vi "Write Configuration.vi"(8 "error in (no error)":errorcluster, 9 "Name (empty: type name)":string, 10 "Type":variant, 11 "ConfigurableActor in":refnum<class "ConfigurableActor.lvclass">) -> (0 "error out":errorcluster, 3 "ConfigurableActor out":refnum<class "ConfigurableActor.lvclass">)   [LabVIEW 2014, in "ConfigurableActor.lvclass"]
uses:
  ConfigurableActor.lvclass
  ConfigurableActor.lvclass/ConfigurableActor.ctl
  <vilib>/LabVIEW Open Source/Configuration Manager/Manager/ConfigManager.lvclass/ConfigManager.ctl
  <vilib>/LabVIEW Open Source/Configuration Manager/Manager/Write.vi
  <vilib>/LabVIEW Open Source/Configuration Manager/Manager/Read Serializer.vi
  <vilib>/LabVIEW Open Source/Configuration Manager/Manager/Read Encoding.vi
  <vilib>/LabVIEW Open Source/Configuration Manager/Manager/Read Encryption.vi
  <vilib>/LabVIEW Open Source/Configuration Manager/Manager/Decompose KVPs.vi
  <vilib>/Utility/VariantDataType/GetTypeInfo.vi
  <vilib>/LabVIEW Open Source/Configuration Manager/Cache/ConfigManager.Cache.lvclass
  <vilib>/LabVIEW Open Source/Configuration Manager/Manager/ConfigManager.lvclass
  <vilib>/LabVIEW Open Source/Configuration Manager/Serializer/Serializer.lvclass
  <vilib>/LabVIEW Open Source/Configuration Manager/Encoding/Encoding.lvclass
  <vilib>/LabVIEW Open Source/Configuration Manager/Encryption/Encryption.lvclass
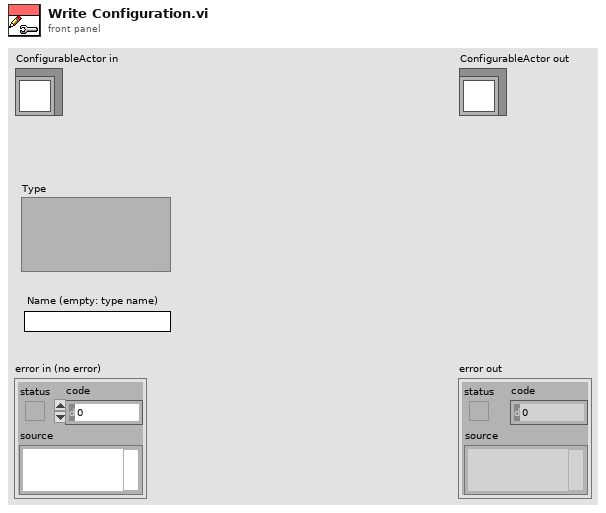
[diagram p1: front panel]
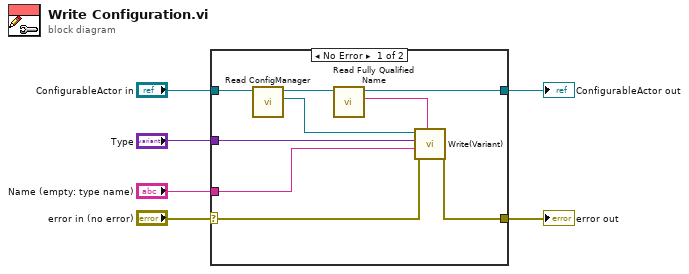
[diagram p0: block diagram]
diagram:
  n1 = case shown="No Error" "error in (no error)" {
    selector: "error in (no error)" -> [w7 w17]
    tunnel: [w8 w17] -> w5
    tunnel: [w13 w16] -> w3
    tunnel: "ConfigurableActor in" -> [w15 w16]
    tunnel: "Type" -> [w12 _]
    tunnel: "Name (empty: type name)" -> [w11 _]
    frame No Error {
      n2 = call "Read ConfigManager.vi"("ConfigurableActor in"=w15) -> ("ConfigManager"=w9:refnum<class "ConfigManager.lvclass">, "ConfigurableActor out"=w14:refnum<class "ConfigurableActor.lvclass">)  [unwired: 8 in, 1 out]
      n3 = call "Read Fully Qualified Name.vi"("ConfigurableActor in"=w14) -> ("Fully Qualified Name"=w10:string, "ConfigurableActor out"=w13:refnum<class "ConfigurableActor.lvclass">)  [unwired: 8 in, 1 out]
      n4 = call <vilib>:"Write(Variant).vi"("Qualified Name"=w10, "error in (no error)"=w7, "Name (empty: va;ue name)"=w11, "value"=w12, "ConfigManager in"=w9) -> ("error out"=w8:errorcluster)  [unwired: 4 in, 2 out]
    }
    frame Error {
    }
  }
  "error out" <- w5
  "ConfigurableActor out" <- w3
